vi "Init SPI.vi"(5 "Data Bits":i8=8, 7 "Mode":T1, 8 "error in (no error)":errorcluster, 9 "Baud":u32=1000000 format="%.0p", 10 "SPI In":refnum<class "SPI.lvclass">, 11 "Session in":refnum<class "Session.lvclass">) -> (0 "error out":errorcluster, 2 "SPI":refnum<class "SPI.lvclass">, 3 "Session out":refnum<class "Session.lvclass">)   [LabVIEW 2020, in "CTI.lvlib" / "Session.lvclass"]
uses:
  Session.lvclass
  SPI/SPI.lvclass
  SPI Mode.ctl
  SPI Config.ctl
  SPI Pins.ctl
  GPIO Number.ctl
  DeviceComms/DeviceComms.lvclass
  CTI.lvlib
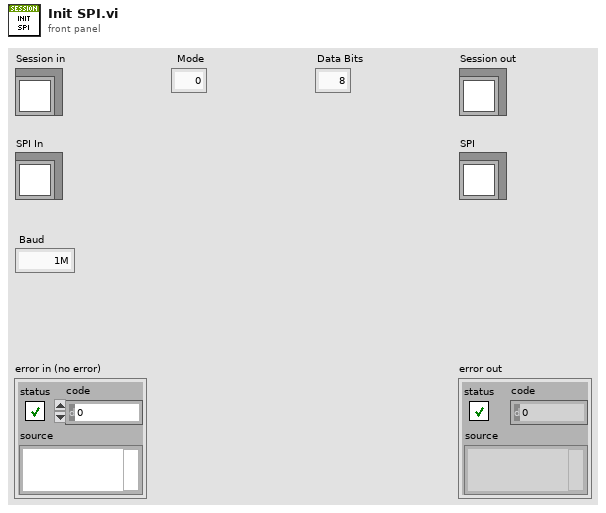
[diagram p1: front panel]
types:
  T1 = typedef "CTI.lvlib/SPI Mode.ctl" = i8
  T2 = typedef "CTI.lvlib/SPI Number.ctl" = i8
  T3 = typedef "CTI.lvlib/GPIO Number.ctl" = i8
  T4 = typedef "CTI.lvlib/SPI Config.ctl" = cluster{"Mode":T1, "Data Bits":i8, "Pins":T5}
  T5 = typedef "CTI.lvlib/SPI Pins.ctl" = cluster{"TX GPIO":T3, "RX GPIO":T3, "SCK GPIO":T3}
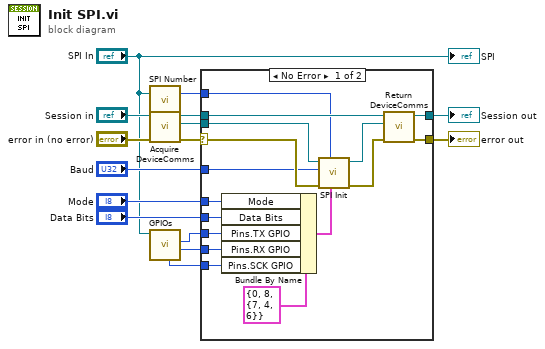
[diagram p0: block diagram]
diagram:
  n1 = call "SPI Number.vi"("SPI in"="SPI In") -> ("SPI #"=w5:T2)  [unwired: 6 in]
  n2 = call "Acquire DeviceComms.vi"("error in (no error)"="error in (no error)", "Session in"="Session in") -> ("error out"=w15:errorcluster, "DeviceComms"=w9:refnum<class "DeviceComms.lvclass">, "Session out"=w7:refnum<class "Session.lvclass">)  [unwired: 7 in]
  n3 = call "GPIOs.vi"("SPI in"="SPI In") -> ("RX GPIO"=w2:T3, "TX GPIO"=w3:T3, "SCK GPIO"=w1:T3)  [unwired: 6 in, 2 out]
  n4 = case shown="No Error" w15 {
    selector: w15 -> [w31 w32]
    tunnel: "Mode" -> [w28 _]
    tunnel: "Data Bits" -> [w27 _]
    tunnel: "Baud" -> [w26 _]
    tunnel: w9 -> [w25 _]
    tunnel: [w24 w32] -> w8
    tunnel: w7 -> [w23 w33]
    tunnel: [w22 w33] -> w6
    tunnel: w5 -> [w19 _]
    tunnel: w3 -> [w18 _]
    tunnel: w2 -> [w17 _]
    tunnel: w1 -> [w16 _]
    frame No Error {
      n5 = Bundle By Name(cluster=T4 {"Mode"=0, "Data Bits"=8, "Pins"={"TX GPIO"=7, "RX GPIO"=4, "SCK GPIO"=6}} ("SPI Config"), "Mode"=w28, "Data Bits"=w27, "Pins.TX GPIO"=w18, "Pins.RX GPIO"=w17, "Pins.SCK GPIO"=w16) -> (w29:T4)
      n6 = call-dynamic "SPI Init.vi"("SPI Config"=w29, "SPI #"=w19, "error in (no error)"=w31, "Baud"=w26, "DeviceComms in"=w25) -> ("error out"=w21:errorcluster, "DeviceComms out"=w20:refnum<class "DeviceComms.lvclass">)  [unwired: 5 in]
      n7 = call "Return DeviceComms.vi"("error in (no error)"=w21, "DeviceComms"=w20, "Session in"=w23) -> ("error out"=w24:errorcluster, "Session out"=w22:refnum<class "Session.lvclass">)  [unwired: 7 in]
    }
    frame Error {
    }
  }
  "error out" <- w8
  "Session out" <- w6
  "SPI" <- "SPI In"
